vi "DeterminePingCommand.vi"() -> (0 "String":string)   [LabVIEW 2018]
uses:
  CurrentSwitchValues_GlobalVariable.vi
panel:
  out "Units 1/2":u8 format="%x"
  out "Units 3/4":u8 format="%x"
  out "Units 5/6":u8 format="%x"
  out "Units 7/8":u8 format="%x"
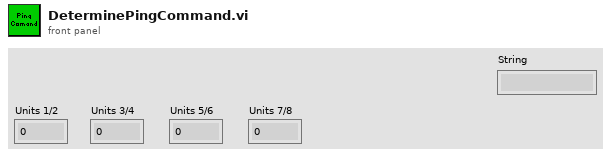
[diagram p1: front panel]
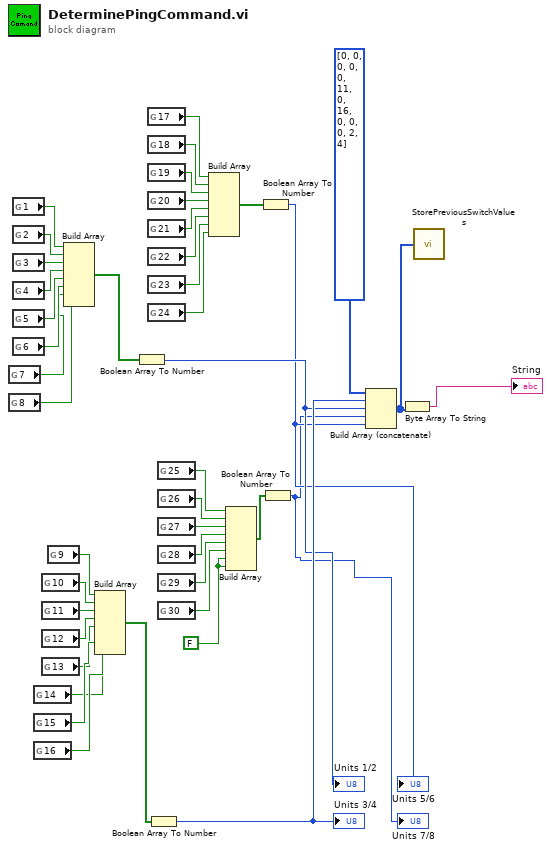
[diagram p0: block diagram]
diagram:
  w1 = FALSE
  n1 = global read "CurrentSwitchValues_GlobalVariable.vi" "7"() -> (w26:bool)
  n2 = global read "CurrentSwitchValues_GlobalVariable.vi" "8"() -> (w25:bool)
  n3 = global read "CurrentSwitchValues_GlobalVariable.vi" "1"() -> (w32:bool)
  n4 = global read "CurrentSwitchValues_GlobalVariable.vi" "2"() -> (w31:bool)
  n5 = global read "CurrentSwitchValues_GlobalVariable.vi" "3"() -> (w30:bool)
  n6 = global read "CurrentSwitchValues_GlobalVariable.vi" "4"() -> (w29:bool)
  n7 = global read "CurrentSwitchValues_GlobalVariable.vi" "5"() -> (w28:bool)
  n8 = global read "CurrentSwitchValues_GlobalVariable.vi" "6"() -> (w27:bool)
  n9 = global read "CurrentSwitchValues_GlobalVariable.vi" "14"() -> (w22:bool)
  n10 = global read "CurrentSwitchValues_GlobalVariable.vi" "15"() -> (w23:bool)
  n11 = global read "CurrentSwitchValues_GlobalVariable.vi" "16"() -> (w24:bool)
  n12 = global read "CurrentSwitchValues_GlobalVariable.vi" "10"() -> (w18:bool)
  n13 = global read "CurrentSwitchValues_GlobalVariable.vi" "11"() -> (w19:bool)
  n14 = global read "CurrentSwitchValues_GlobalVariable.vi" "12"() -> (w20:bool)
  n15 = global read "CurrentSwitchValues_GlobalVariable.vi" "13"() -> (w21:bool)
  n16 = global read "CurrentSwitchValues_GlobalVariable.vi" "9"() -> (w17:bool)
  n17 = Build Array "Build Array"(w32, w31, w30, w29, w28, w27, w26, w25) -> (w33:bool[])
  n18 = Build Array "Build Array"(w17, w18, w19, w20, w21, w22, w23, w24) -> (w34:bool[])
  n19 = Boolean Array To Number(Boolean array=w33) -> (number=w40:u32)
  "Units 1/2" <- w40
  n20 = global read "CurrentSwitchValues_GlobalVariable.vi" "17"() -> (w5:bool)
  n21 = global read "CurrentSwitchValues_GlobalVariable.vi" "18"() -> (w4:bool)
  n22 = global read "CurrentSwitchValues_GlobalVariable.vi" "19"() -> (w3:bool)
  n23 = global read "CurrentSwitchValues_GlobalVariable.vi" "20"() -> (w10:bool)
  n24 = global read "CurrentSwitchValues_GlobalVariable.vi" "21"() -> (w9:bool)
  n25 = global read "CurrentSwitchValues_GlobalVariable.vi" "22"() -> (w8:bool)
  n26 = global read "CurrentSwitchValues_GlobalVariable.vi" "23"() -> (w7:bool)
  n27 = global read "CurrentSwitchValues_GlobalVariable.vi" "24"() -> (w6:bool)
  n28 = Boolean Array To Number(Boolean array=w34) -> (number=w41:u32)
  "Units 3/4" <- w41
  n29 = global read "CurrentSwitchValues_GlobalVariable.vi" "25"() -> (w11:bool)
  n30 = global read "CurrentSwitchValues_GlobalVariable.vi" "26"() -> (w12:bool)
  n31 = global read "CurrentSwitchValues_GlobalVariable.vi" "27"() -> (w13:bool)
  n32 = global read "CurrentSwitchValues_GlobalVariable.vi" "28"() -> (w14:bool)
  n33 = global read "CurrentSwitchValues_GlobalVariable.vi" "29"() -> (w15:bool)
  n34 = global read "CurrentSwitchValues_GlobalVariable.vi" "30"() -> (w16:bool)
  n35 = Build Array "Build Array"(w5, w4, w3, w10, w9, w8, w7, w6) -> (w35:bool[])
  n36 = Build Array "Build Array"(w11, w12, w13, w14, w15, w16, w1, w1) -> (w36:bool[])
  n37 = Boolean Array To Number(Boolean array=w35) -> (number=w39:u32)
  "Units 5/6" <- w39
  n38 = Boolean Array To Number(Boolean array=w36) -> (number=w38:u32)
  "Units 7/8" <- w38
  n39 = Build Array (concatenate)(u8[] [0, 0, 0, 0, 0, 11, 0, 16, 0, 0, 0, 2, 4], w41, w40, w38, w39) -> (w42:u32[])
  n40 = Byte Array To String(unsigned byte array=w42) -> (string=→"String":string)
  n41 = call "StorePreviousSwitchValues.vi"("Array"=w42) -> ()  [unwired: 3 in]
